vi "Get Registry.vi"() -> (3 "Registry":refnum<data-value>)   [LabVIEW 2014, in "ConfigurableQMH.lvlib"]
uses:
  <vilib>/LabVIEW Open Source Project/Unicity/UniqueName/Registry/NameRegistry.lvclass
  ConfigurableQMH.lvlib
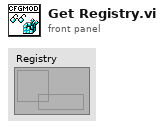
[diagram p1: front panel]
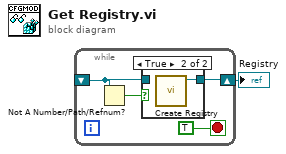
[diagram p0: block diagram]
diagram:
  n1 = while {
    shift-right: [w4] -> w1
    shift-left: _ -> [w2]
    stop <- TRUE stop-if-true
    n2 = Not A Number/Path/Refnum?(number/path/refnum=w2) -> (NaN/Path/Refnum?=w3:bool)
    n3 = case shown="True" w3 {
      tunnel: [w6 w7] -> w4
      tunnel: w2 -> [w6 _]
      frame False {
      }
      frame True {
        n4 = call <vilib>:"Create Registry.vi"() -> ("Registry"=w7:refnum<data-value>)  [unwired: 10 in, 1 out]
      }
    }
  }
  "Registry" <- w1
